vi "Clear-sequences-UI.vi"(8 "error in (no error)":errorcluster, 11 "Object ref in":T1) -> (0 "error out":errorcluster, 3 "Object ref out":T1)   [LabVIEW 2013, in "PowderDeposition.lvlib" / "PD-Main.lvclass"]
uses:
  PD-Main.lvclass
  Object-reference.ctl
  PD-Main.lvclass/PD-Main.ctl
  Read Motor sequences.vi
  Assembly/Motor-assembly.lvclass
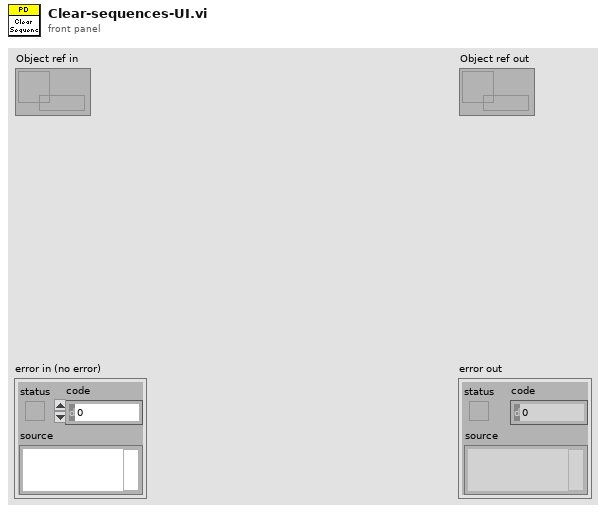
[diagram p1: front panel]
types:
  T1 = typedef "PowderDeposition.lvlib/PD-Main.lvclass/Object-reference.ctl" = refnum<data-value>
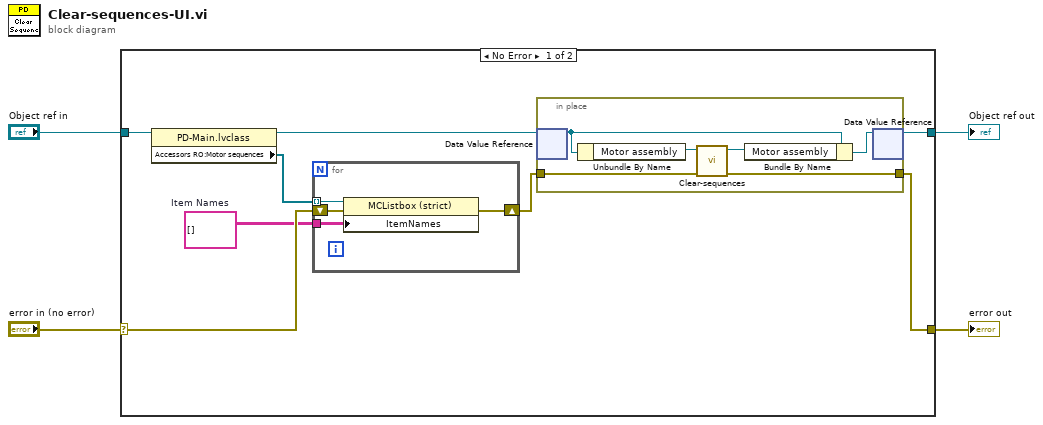
[diagram p0: block diagram]
diagram:
  n1 = case shown="No Error" "error in (no error)" {
    selector: "error in (no error)" -> [w11 w24]
    tunnel: [w5 w24] -> w3
    tunnel: [w7 w23] -> w1
    tunnel: "Object ref in" -> [w12 w23]
    frame No Error {
      w10 = string[][] []  # Item Names
      n2 = property class="PD-Main.lvclass"(reference=w12) -> (reference out=w8:T1, "Accessors RO:Motor sequences"=w9:refnum<vi>[])  [unwired: 1 in, 1 out]
      n3 = for {
        tunnel: w10 -> [w20]
        tunnel: w9 -> [w19] mode=indexing
        shift-right: [w22] -> w6
        shift-left: w11 -> [w21]
        n4 = property class="MCListbox (strict)"(reference=w19, error in=w21, "ItemNames"=w20) -> (error out=w22:errorcluster)  [unwired: 1 out]
      }
      n5 = in-place {
        in-place-border: w6 -> [w17]
        in-place-border: [w13] -> w5
        n6 = in-place-dvr #1(w8) -> (w15:refnum<class "PD-Main.lvclass">)  [unwired: 1 out]
        n7 = Unbundle By Name(w15) -> ("Motor assembly"=w18:refnum<class "Motor-assembly.lvclass">)
        n8 = call "Clear-sequences.vi"("error in (no error)"=w17, "Available motors in"=w18) -> ("error out"=w13:errorcluster, "Available motors out"=w16:refnum<class "Motor-assembly.lvclass">)  [unwired: 8 in]
        n9 = Bundle By Name(cluster=w15, "Motor assembly"=w16) -> (w14:refnum<class "PD-Main.lvclass">)
        n10 = in-place-dvr #1(w14) -> (w7:T1)  [unwired: 1 out]
      }
    }
    frame Error {
    }
  }
  "error out" <- w3
  "Object ref out" <- w1
